vi "Stop FGV.vi"(6 "Enum":T1, 8 "error in (no error)":errorcluster) -> (0 "error out":errorcluster, 2 "Stop":refnum<user-event>, 3 "Event Registration Refnum":refnum<event-registration>)   [LabVIEW 2018]
uses:
  Controles/FGV Opciones.ctl
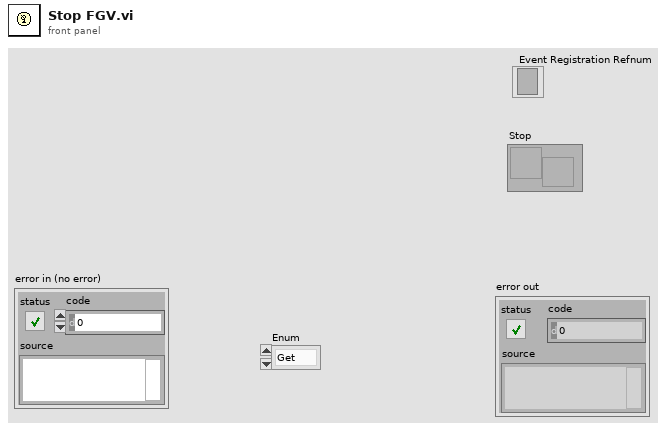
[diagram p1: front panel]
types:
  T1 = typedef "FGV Opciones.ctl" = enum16{"Get", "Create", "Destroy"}
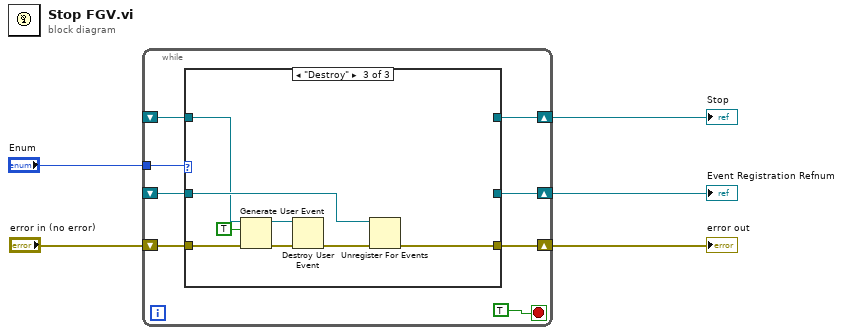
[diagram p0: block diagram]
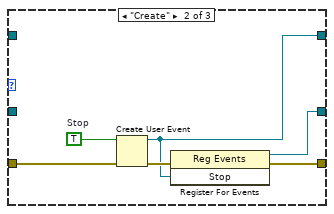
[diagram p3: hidden frame]
diagram:
  n1 = while {
    tunnel: "Enum" -> [w11]
    shift-right: [w12] -> w4
    shift-left: "error in (no error)" -> [w13]
    shift-right: [w8] -> w1
    shift-left: _ -> [w6]
    shift-right: [w9] -> w2
    shift-left: _ -> [w7]
    stop <- TRUE stop-if-true
    n2 = case shown="\"Destroy\"" w11 {
      tunnel: w13 -> [w14 w21 w25]
      tunnel: [w14 w20 w24] -> w12
      tunnel: [w15 w18 _] -> w9
      tunnel: [w16 w17 _] -> w8
      tunnel: w7 -> [w15 _ w30]
      tunnel: w6 -> [w16 _ w29]
      frame "Get", Default {
      }
      frame "Create" {
        w19 = TRUE  # Stop
        n3 = Create User Event(user event datatype=w19, error in=w21) -> (user event=w17:refnum<user-event>, error out=w22:errorcluster)
        n4 = register-events(error in=w22, w17) -> (reference out=w18:refnum<event-registration>, error out=w20:errorcluster)  [unwired: 1 in]
      }
      frame "Destroy" {
        n5 = Generate User Event(user event=w29, event data cluster=TRUE ("event data"), error in=w25) -> (user event out=w28:refnum<user-event>, error out=w27:errorcluster)  [unwired: 1 in]
        n6 = Destroy User Event(user event=w28, error in=w27) -> (error out=w26:errorcluster)
        n7 = Unregister For Events(event registration refnum=w30, error in=w26) -> (error out=w24:errorcluster)
      }
    }
  }
  "error out" <- w4
  "Event Registration Refnum" <- w2
  "Stop" <- w1
